vi "IDE Util.Manage Exec VIs.vi"() -> ()   [LabVIEW 2018]
panel:
  in  "Main Tab":enum32{"Operate", "Maint"}(tab)
  in  "Deselect All":bool
  in  "Select All":bool
  in  "Abort":bool
  in  "Abort VIs":bool
  in  "Show VIs":bool
  in  "Get VIs":bool
  in  "VI List":i32[](listbox)
  in  "Execution:State":T1(ring)=enum."Run top level"
  in  "Exit And Close":bool
  # "VI Manager"
  # "Lists only open and/or executing VIs"
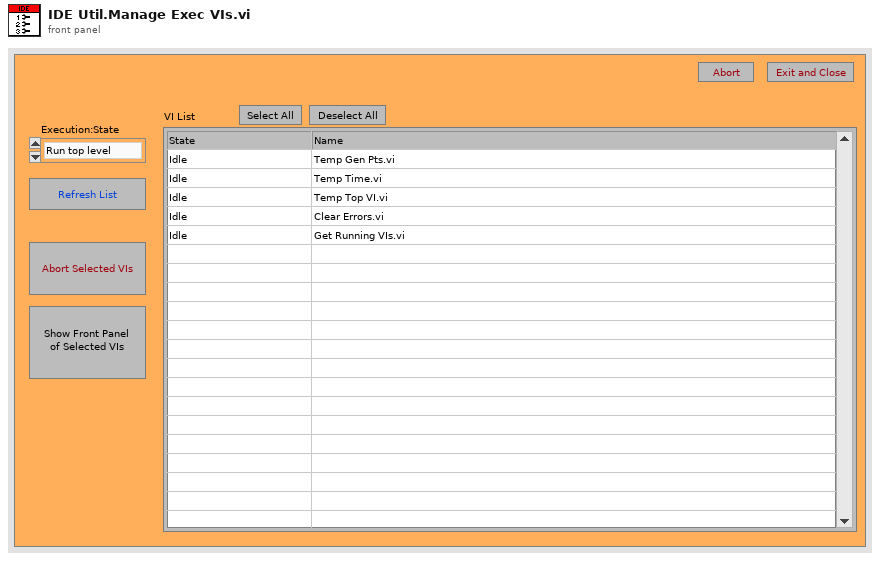
[diagram p1: front panel]
types:
  T1 = enum32{"Bad", "Idle", "Run top level", "Running"}
  T2 = enum32{"Invalid", "Standard", "Closed", "Hidden", "Minimized", "Maximized"}
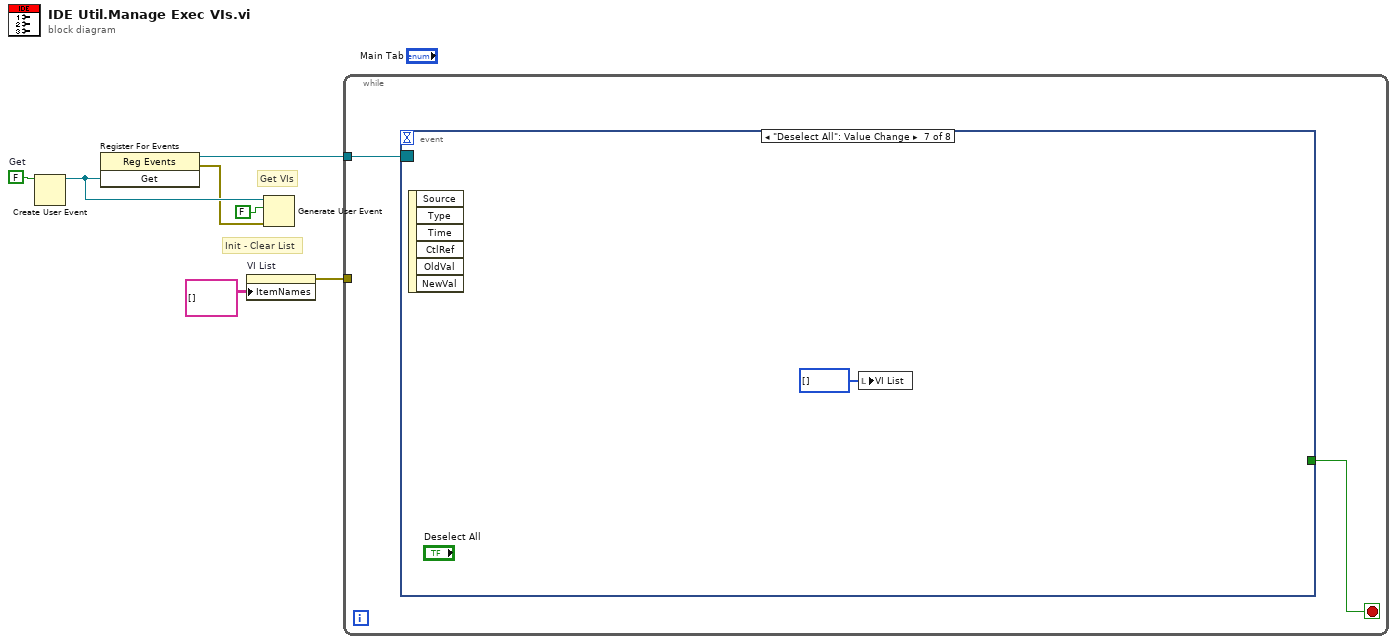
[diagram p0: block diagram]
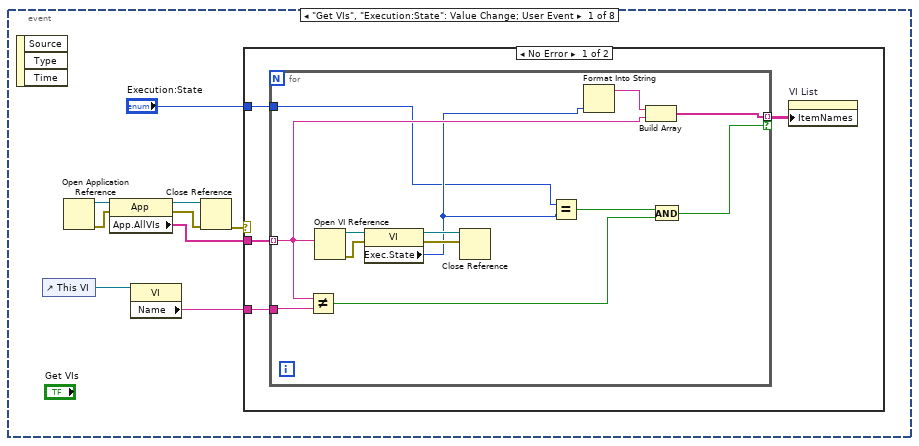
[diagram p2: hidden frame]
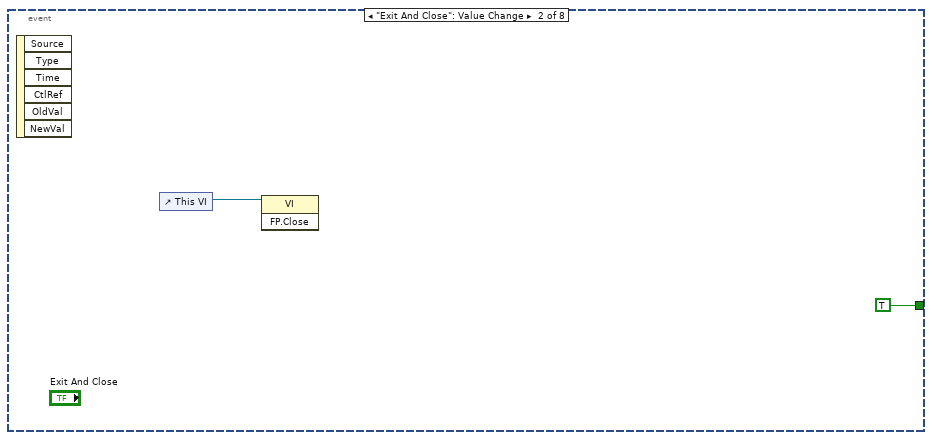
[diagram p4: hidden frame]
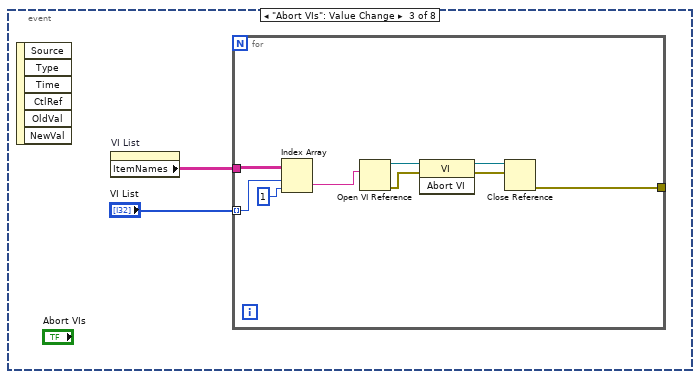
[diagram p5: hidden frame]
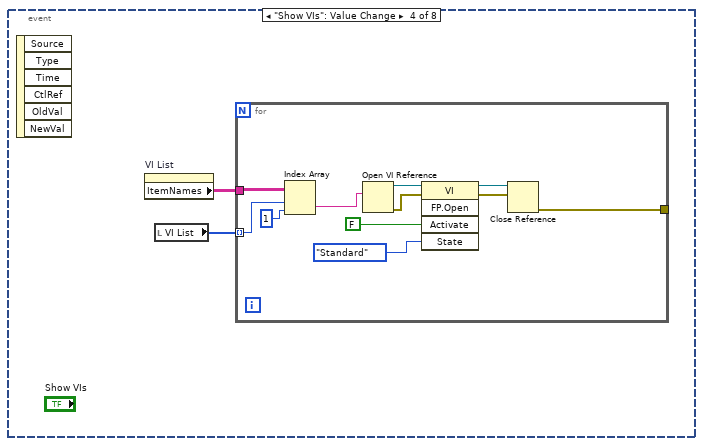
[diagram p6: hidden frame]
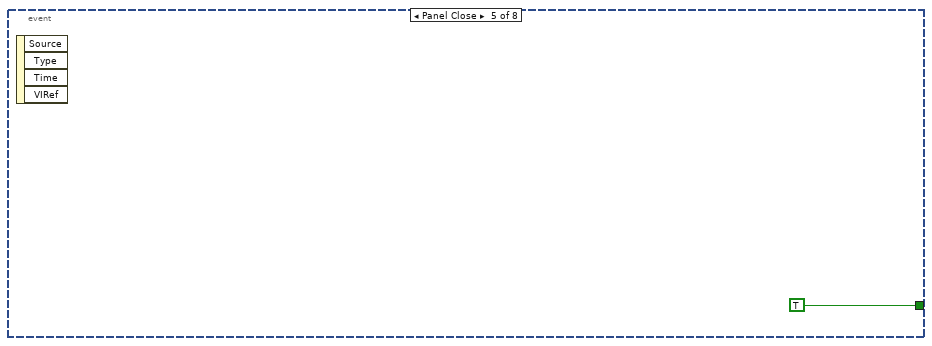
[diagram p7: hidden frame]
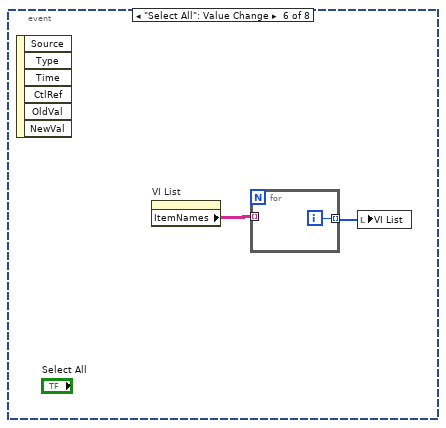
[diagram p8: hidden frame]
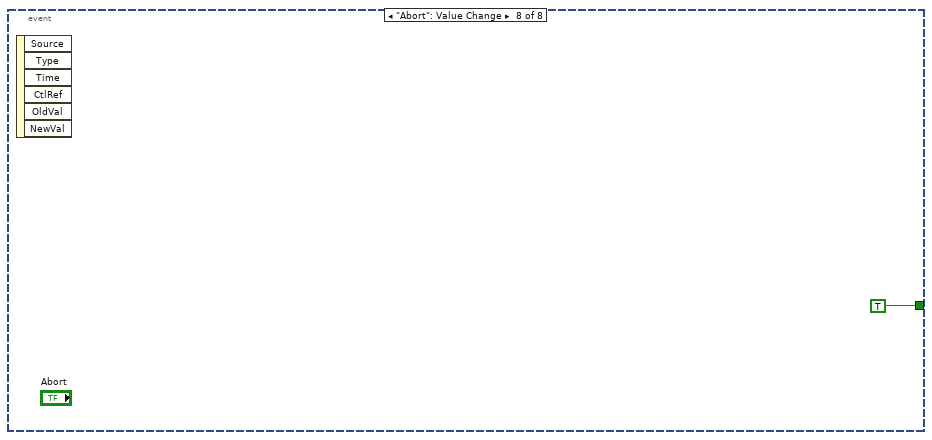
[diagram p9: hidden frame]
diagram:
  w4 = FALSE  # Get
  # "Get VIs"
  # "Init - Clear List"
  n1 = Create User Event(user event datatype=w4) -> (user event=w3:refnum<user-event>)  [unwired: 1 in, 1 out]
  n2 = register-events(w3) -> (reference out=w5:refnum<event-registration>, error out=w1:errorcluster)  [unwired: 2 in]
  n3 = property on="VI List" class="MCListbox (strict)"("ItemNames"=string[][] [] ("Item Names")) -> (error out=w6:errorcluster)  [unwired: 2 in, 1 out]
  n4 = Generate User Event(user event=w3, event data cluster=FALSE ("event data"), error in=w1) -> ()  [unwired: 1 in, 2 out]
  n5 = while {
    tunnel: w6 -> [_]
    tunnel: w5 -> [w8]
    stop <- w9 stop-if-true
    n6 = event shown="[6] \"Deselect All\": Value Change" {
      selector: w8 -> [_ _ _ _ _ _ _ _]
      dyn-events: _ -> [_ _ _ _ _ _ _ _]
      timeout: _ -> [_ _ _ _ _ _ _ _]
      tunnel: [_ TRUE _ _ TRUE _ _ TRUE] -> w9
      event "Get VIs", "Execution:State": Value Change; User Event {
        n7 = event-data() -> ()  [unwired: 1 in, 3 out]
        n8 = control-ref of="This VI"() -> (w11:refnum<vi>)
        n9 = Open Application Reference() -> (0:w16:errorcluster, 3:w12:refnum<vi>)  [unwired: 4 in]
        n10 = property class="App"(reference=w12, error in=w16) -> (reference out=w13:refnum<vi>, error out=w17:errorcluster, "App.AllVIs"=w15:string[])
        n11 = property class="VI"(reference=w11) -> ("Name"=w10:string)  [unwired: 1 in, 2 out]
        n12 = Close Reference(reference=w13, error in (no error)=w17) -> (error out=w14:errorcluster)
        n13 = case shown="No Error" w14 {
          tunnel: w15 -> [w22 _]
          tunnel: "Execution:State" -> [w20 _]
          tunnel: w10 -> [w19 _]
          frame No Error {
            n14 = for {
              tunnel: w22 -> [w28] mode=indexing
              tunnel: [w30] -> w21 mode=indexing if=w27
              tunnel: w20 -> [w24]
              tunnel: w19 -> [w29]
              n15 = Not Equal?(x=w28, y=w29) -> (x != y?=w26:bool)
              n16 = Open VI Reference(vi path=w28) -> (vi reference=w33:refnum<vi>, error out=w32:errorcluster)  [unwired: 5 in]
              n17 = property class="VI"(reference=w33, error in=w32) -> (reference out=w35:refnum<vi>, error out=w34:errorcluster, "Exec.State"=w25:T1)
              n18 = Close Reference(reference=w35, error in (no error)=w34) -> ()  [unwired: 1 out]
              n19 = Equal?(x=w24, y=w25) -> (x = y?=w23:bool)
              n20 = Format Into String(w25) -> (resulting string=w31:string)  [unwired: 3 in, 1 out]
              n21 = Build Array(w31, w28) -> (w30:string[])
              n22 = And(x=w23, y=w26) -> (x .and. y?=w27:bool)
            }
            n23 = property on="VI List" class="MCListbox (strict)"("ItemNames"=w21) -> ()  [unwired: 2 in, 2 out]
          }
          frame Error {
          }
        }
      }
      event "Exit And Close": Value Change {
        n24 = event-data() -> ()  [unwired: 1 in, 6 out]
        n25 = control-ref of="This VI"() -> (w36:refnum<vi>)
        n26 = invoke class="VI" method="FP.Close"(reference=w36) -> ()  [unwired: 2 in, 3 out]
      }
      event "Abort VIs": Value Change {
        n27 = event-data() -> ()  [unwired: 1 in, 6 out]
        n28 = property on="VI List" class="MCListbox (strict)"() -> ("ItemNames"=w38:string[][])  [unwired: 2 in, 2 out]
        n29 = for {
          tunnel: "VI List" -> [w47] mode=indexing
          tunnel: w38 -> [w48]
          tunnel: [w40] -> _
          n30 = Index Array(array=w48, index (row)=w47, index (col)=1 ("disabled index (col)")) -> (element=w41:string)
          n31 = Open VI Reference(vi path=w41) -> (vi reference=w43:refnum<vi>, error out=w42:errorcluster)  [unwired: 5 in]
          n32 = invoke class="VI" method="Abort VI"(reference=w43, error in=w42) -> (reference out=w45:refnum<vi>, error out=w44:errorcluster)  [unwired: 1 in, 1 out]
          n33 = Close Reference(reference=w45, error in (no error)=w44) -> (error out=w40:errorcluster)
        }
      }
      event "Show VIs": Value Change {
        n34 = event-data() -> ()  [unwired: 1 in, 6 out]
        n35 = property on="VI List" class="MCListbox (strict)"() -> ("ItemNames"=w50:string[][])  [unwired: 2 in, 2 out]
        n36 = local read "VI List"() -> (w49:i32[])
        n37 = for {
          tunnel: w49 -> [w60] mode=indexing
          tunnel: w50 -> [w61]
          tunnel: [w53] -> _
          n38 = Index Array(array=w61, index (row)=w60, index (col)=1 ("disabled index (col)")) -> (element=w54:string)
          n39 = Open VI Reference(vi path=w54) -> (vi reference=w56:refnum<vi>, error out=w55:errorcluster)  [unwired: 5 in]
          n40 = invoke class="VI" method="FP.Open"(reference=w56, error in=w55, "Activate"=FALSE ("Activate?"), "State"=T2."Standard") -> (reference out=w58:refnum<vi>, error out=w57:errorcluster)  [unwired: 1 in, 3 out]
          n41 = Close Reference(reference=w58, error in (no error)=w57) -> (error out=w53:errorcluster)
        }
      }
      event Panel Close {
        n42 = event-data() -> ()  [unwired: 1 in, 4 out]
      }
      event "Select All": Value Change {
        n43 = event-data() -> ()  [unwired: 1 in, 6 out]
        n44 = property on="VI List" class="MCListbox (strict)"() -> ("ItemNames"=w64:string[][])  [unwired: 2 in, 2 out]
        n45 = for {
          tunnel: w64 -> [_] mode=indexing
          tunnel: [w65] -> w63 mode=indexing
          i -> [w65]
        }
        n46 = local write "VI List"(w63) -> ()
      }
      event "Deselect All": Value Change {
        n47 = event-data() -> ()  [unwired: 1 in, 6 out]
        n48 = local write "VI List"(i32[] [] ("VI List")) -> ()
      }
      event "Abort": Value Change {
        n49 = event-data() -> ()  [unwired: 1 in, 6 out]
      }
    }
  }
